vi "P1E1 RLJ 2015640305.vi"() -> ()   [LabVIEW 2016]
panel:
  in  "X2":bool
  in  "X1":bool
  out "XNOR":bool
  out "XOR":bool
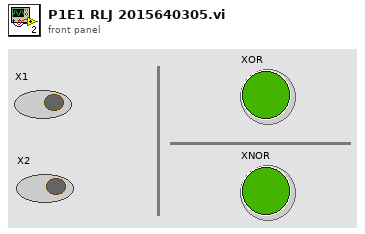
[diagram p1: front panel]
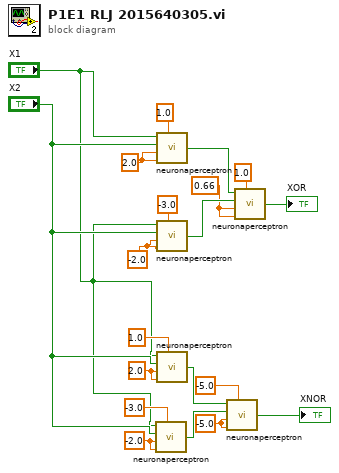
[diagram p0: block diagram]
diagram:
  w6 = -5.0 ("w 1")
  w10 = 2.0 ("w 1")
  w11 = -2.0 ("w 1")
  w14 = 0.66 ("w 1")
  w18 = 2.0 ("w 1")
  w19 = -2.0 ("w 1")
  n1 = call "neuronaperceptron.vi"("X1"="X1", "X2"="X2", "w 1"=w11, "w 2"=w11, "B"=-3.0) -> ("A"=w7:bool)
  n2 = call "neuronaperceptron.vi"("X1"="X1", "X2"="X2", "w 1"=w18, "w 2"=w18, "B"=1.0) -> ("A"=w16:bool)
  n3 = call "neuronaperceptron.vi"("X1"="X1", "X2"="X2", "w 1"=w19, "w 2"=w19, "B"=-3.0) -> ("A"=w15:bool)
  n4 = call "neuronaperceptron.vi"("X1"="X1", "X2"="X2", "w 1"=w10, "w 2"=w10, "B"=1.0) -> ("A"=w8:bool)
  n5 = call "neuronaperceptron.vi"("X1"=w8, "X2"=w7, "w 1"=w6, "w 2"=w6, "B"=-5.0) -> ("A"=→"XNOR":bool)
  n6 = call "neuronaperceptron.vi"("X1"=w16, "X2"=w15, "w 1"=w14, "w 2"=w14, "B"=1.0) -> ("A"=→"XOR":bool)
